vi "STATISTICAL ANALYSIS.vi"() -> ()   [LabVIEW 2019]
uses:
  <vilib>/Analysis/baseanly.llb/Mean (DBL).vi
  <vilib>/Analysis/baseanly.llb/Unimode.vi
  <vilib>/Analysis/NI_AALPro.lvlib
  <vilib>/Analysis/NI_AALBase.lvlib
panel:
  out "array of clusters":cluster{"Time Delta":dynamicdata}[](array[cluster])
  out "mode":dbl
  out "variance":dbl format="%0.2f"
  out "standard deviation":dbl format="%0.2f"
  out "mean 2":dbl format="%0.2f"
  out "mean":dbl format="%0.2f"
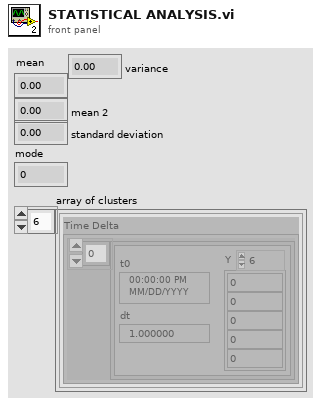
[diagram p1: front panel]
types:
  T1 = enum16{"sine", "cosine", "triangle", "square", "sawtooth", "increasing ramp", "decreasing ramp"}
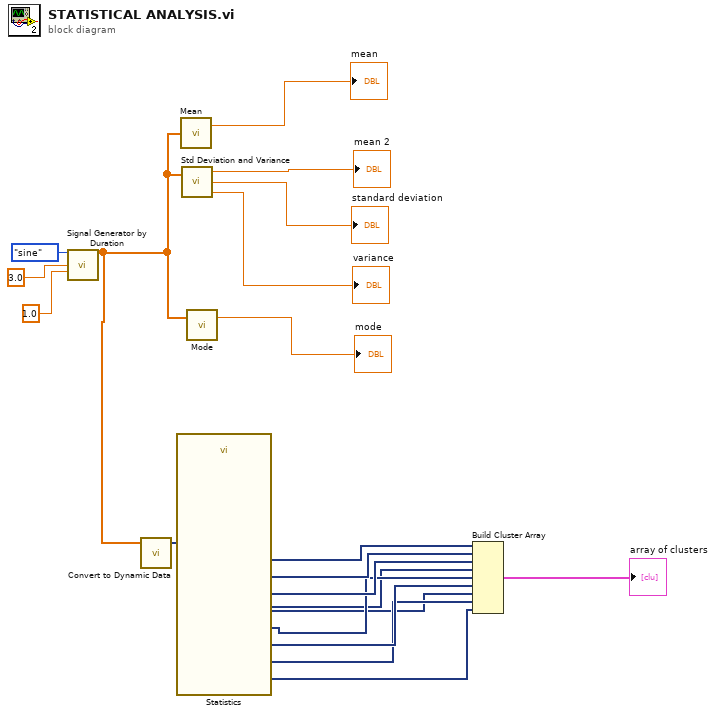
[diagram p0: block diagram]
diagram:
  n1 = call <vilib>:"Signal Generator by Duration.vi"("signal type"=T1."sine", "frequency"=3.0, "amplitude"=1.0) -> ("signal"=w11:dbl[])  [unwired: 9 in, 3 out]
  n2 = call "Convert to Dynamic Data"("Array"=w11) -> ("Dynamic Data Type"=w10:dynamicdata)  [unwired: 3 in]
  n3 = call "Statistics"("Signals"=w10) -> ("Total Samples"=w4:dynamicdata, "Median"=w1:dynamicdata, "Standard Dev"=w7:dynamicdata, "RMS"=w8:dynamicdata, "Arithmetic Mean"=w9:dynamicdata, "Time Delta"=w3:dynamicdata, "Minimum"=w5:dynamicdata, "Maximum"=w6:dynamicdata)  [unwired: 18 in, 1 out]
  n4 = call-poly <vilib>:"Mean.vi"("X"=w11) -> ("mean"=→"mean":dbl)  [unwired: 1 out]
  n5 = call <vilib>:"Std Deviation and Variance.vi"("X"=w11) -> ("mean"=→"mean 2":dbl, "standard deviation"=→"standard deviation":dbl, "variance"=→"variance":dbl)  [unwired: 1 in]
  n6 = call-poly <vilib>:"Mode.vi"("X"=w11) -> ("mode"=→"mode":dbl)  [unwired: 1 in, 1 out]
  n7 = Build Cluster Array(w9, w8, w7, w1, w6, w5, w1, w4, w3) -> (→"array of clusters":cluster{"Time Delta":dynamicdata}[])
